vi "Read All Settings From File.vi"(8 "error in":errorcluster, 11 "Archivist in":refnum<class "Archivist.lvclass">) -> (0 "error out":errorcluster, 3 "Archivist out":refnum<class "Archivist.lvclass">)   [LabVIEW 2019, in "Archivist.lvclass"]
uses:
  Archivist.lvclass
  Settings/Path Settings/Path Settings.lvclass
  Settings/Rectangle Settings/Rectangle Settings.lvclass
  Settings/Funnel Settings/Funnel Settings.lvclass
  C:/Users/Albro/Documents/GitHub/AFM-Lithography/lvsrc/Classes/Settings/ObjectSettings/ObjectSettings.lvclass
panel:
  out "Funnel Settings":refnum<class "Funnel Settings.lvclass">[](array[class])
  out "Rectangle Settings":refnum<class "Rectangle Settings.lvclass">[](array[class])
  out "Path Settings":refnum<class "Path Settings.lvclass">[](array[class])
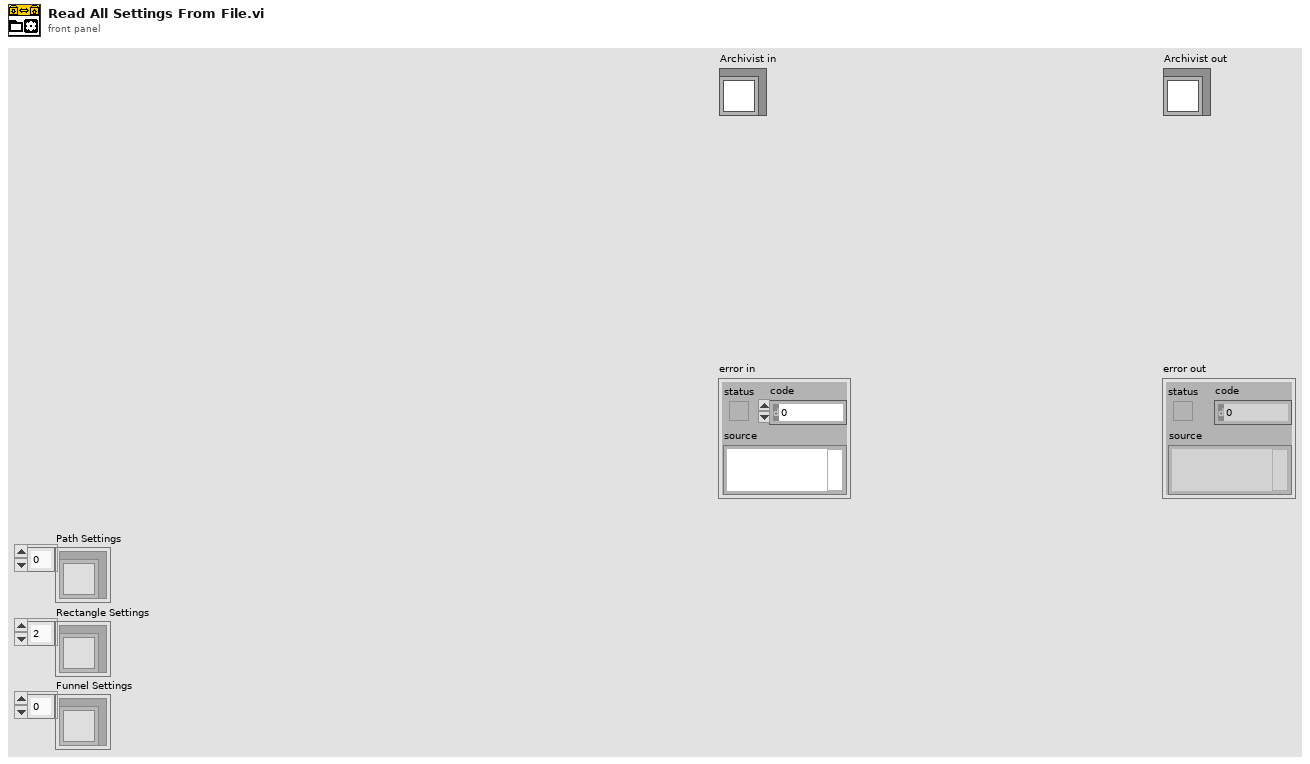
[diagram p1: front panel]
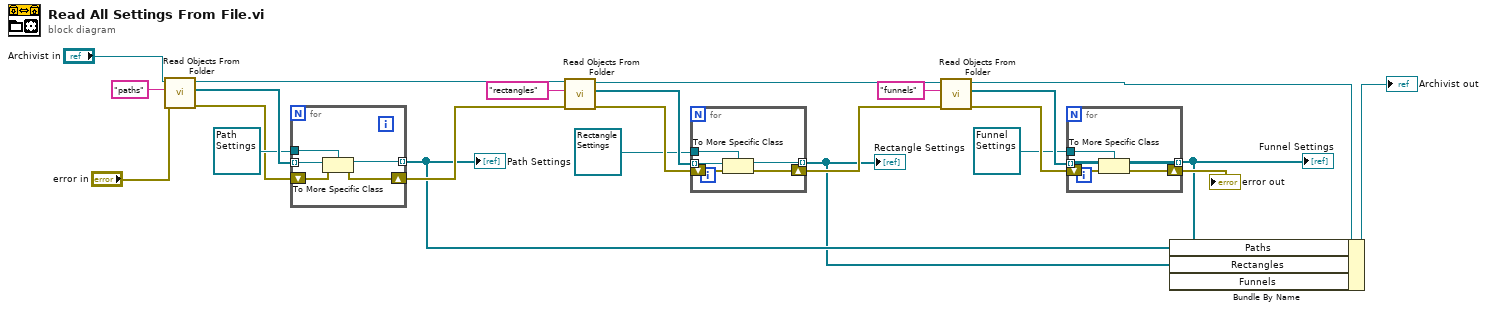
[diagram p0: block diagram]
diagram:
  n1 = call "Read Objects From Folder.vi"("error in"="error in", "Key"="paths", "Archivist in"="Archivist in") -> ("error out"=w21:errorcluster, "Object Settings Array"=w23:refnum<class "ObjectSettings.lvclass">[], "Archivist out"=w6:refnum<class "Archivist.lvclass">)  [unwired: 5 in, 1 out]
  n2 = for {
    tunnel: w23 -> [w29] mode=indexing
    tunnel: refnum<class "Path Settings.lvclass"> refnum ("Path Settings.lvclass") -> [w27]
    tunnel: [w28] -> w3 mode=indexing
    shift-right: [w26] -> w11
    shift-left: w21 -> [w25]
    n3 = To More Specific Class(target class=w27, reference=w29, error in=w25) -> (specific class reference=w28:refnum<class "Path Settings.lvclass">, error out=w26:errorcluster)
  }
  "Path Settings" <- w3
  n4 = call "Read Objects From Folder.vi"("error in"=w11, "Key"="rectangles", "Archivist in"=w6) -> ("error out"=w20:errorcluster, "Object Settings Array"=w19:refnum<class "ObjectSettings.lvclass">[], "Archivist out"=w12:refnum<class "Archivist.lvclass">)  [unwired: 5 in, 1 out]
  n5 = for {
    tunnel: w19 -> [w34] mode=indexing
    tunnel: refnum<class "Rectangle Settings.lvclass"> refnum ("Rectangle Settings.lvclass") -> [w30]
    tunnel: [w33] -> w2 mode=indexing
    shift-right: [w31] -> w10
    shift-left: w20 -> [w32]
    n6 = To More Specific Class(target class=w30, reference=w34, error in=w32) -> (specific class reference=w33:refnum<class "Rectangle Settings.lvclass">, error out=w31:errorcluster)
  }
  "Rectangle Settings" <- w2
  n7 = call "Read Objects From Folder.vi"("error in"=w10, "Key"="funnels", "Archivist in"=w12) -> ("error out"=w14:errorcluster, "Object Settings Array"=w15:refnum<class "ObjectSettings.lvclass">[], "Archivist out"=w5:refnum<class "Archivist.lvclass">)  [unwired: 5 in, 1 out]
  n8 = for {
    tunnel: w15 -> [w39] mode=indexing
    tunnel: refnum<class "Funnel Settings.lvclass"> refnum ("Funnel Settings.lvclass") -> [w35]
    tunnel: [w38] -> w1 mode=indexing
    shift-right: [w36] -> w9
    shift-left: w14 -> [w37]
    n9 = To More Specific Class(target class=w35, reference=w39, error in=w37) -> (specific class reference=w38:refnum<class "Funnel Settings.lvclass">, error out=w36:errorcluster)
  }
  "error out" <- w9
  "Funnel Settings" <- w1
  n10 = Bundle By Name(cluster=w5, "Paths"=w3, "Rectangles"=w2, "Funnels"=w1) -> (→"Archivist out":refnum<class "Archivist.lvclass">)
